vi "Update Message Setter.vi"(7 "RPC Message Name":string, 8 "error in (no error)":errorcluster, 10 "Message Getter in":refnum<vi>, 11 "RPC Messages Folder (ProjectItem) in":refnum<vi>) -> (0 "error out":errorcluster, 2 "Message Getter out":refnum<vi>, 3 "RPC Messages Folder (ProjectItem) out":refnum<vi>)   [LabVIEW 2019, in "gRPC Scripting Tools.lvlib"]
uses:
  gRPC Scripting Tools.lvlib
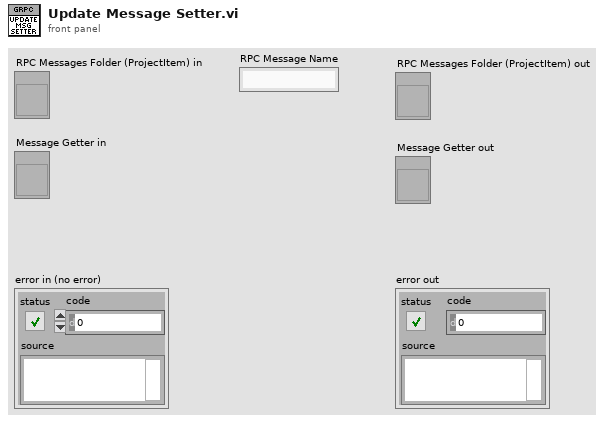
[diagram p1: front panel]
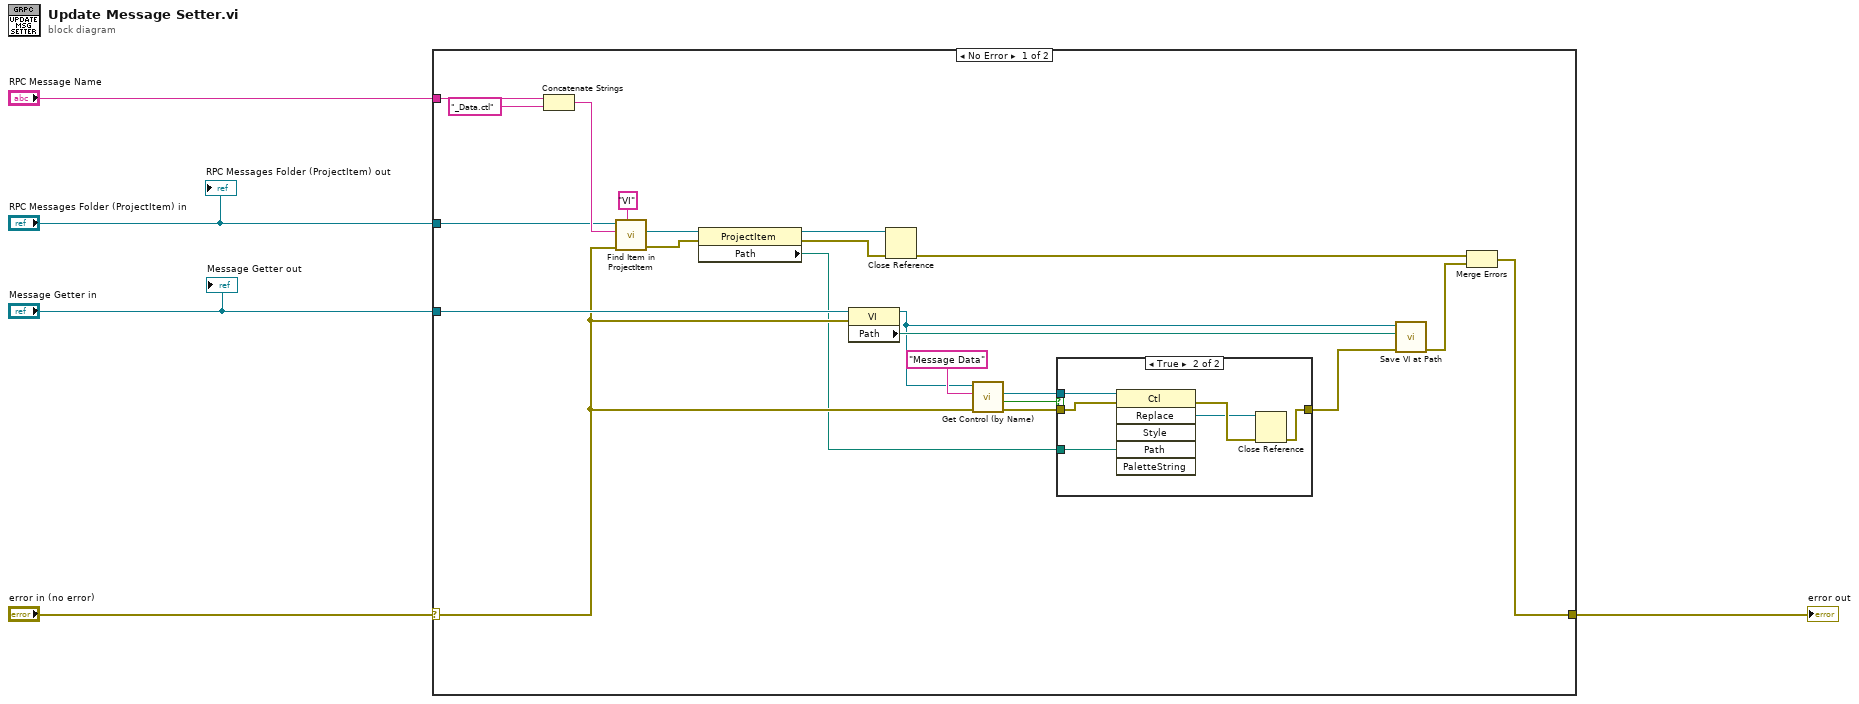
[diagram p0: block diagram]
diagram:
  n1 = case shown="No Error" "error in (no error)" {
    selector: "error in (no error)" -> [w8 w35]
    tunnel: "Message Getter in" -> [w26 _]
    tunnel: [w25 w35] -> w4
    tunnel: "RPC Message Name" -> [w16 _]
    tunnel: "RPC Messages Folder (ProjectItem) in" -> [w14 _]
    frame No Error {
      n2 = Concatenate Strings(w16, "_Data.ctl" ("string")) -> (w18:string)
      n3 = call "Find Item in ProjectItem.vi"("Item Type"="VI", "error in (no error)"=w8, "Name"=w18, "ProjectItem in"=w14) -> ("error out"=w20:errorcluster, "Item Refnum out"=w19:refnum<vi>)  [unwired: 4 in, 2 out]
      n4 = property class="ProjectItem"(reference=w19, error in=w20) -> (reference out=w21:refnum<vi>, error out=w22:errorcluster, "Path"=w6:path)
      n5 = property class="VI"(reference=w26, error in=w8) -> (reference out=w9:refnum<vi>, "Path"=w27:path)  [unwired: 1 out]
      n6 = Close Reference(reference=w21, error in (no error)=w22) -> (error out=w24:errorcluster)
      n7 = call "Get Control (by Name).vi"("error in (no error)"=w8, "Control Label"="Message Data" ("name/order"), "Owner VI in"=w9) -> ("error out"=w12:errorcluster, "Found ?"=w13:bool, "Control Refnum"=w11:refnum<vi>)  [unwired: 5 in, 1 out]
      n8 = case shown="True" w13 {
        tunnel: [w28 w34] -> w7
        tunnel: w11 -> [_ w31]
        tunnel: w12 -> [w28 w30]
        tunnel: w6 -> [_ w29]
        frame False {
        }
        frame True {
          n9 = invoke class="Ctl" method="Replace"(reference=w31, error in=w30, "Path"=w29) -> (error out=w33:errorcluster, "Replace"=w32:refnum<vi>)  [unwired: 3 in, 4 out]
          n10 = Close Reference(reference=w32, error in (no error)=w33) -> (error out=w34:errorcluster)
        }
      }
      n11 = call "Save VI at Path.vi"("error in (no error)"=w7, "Path"=w27, "VI in"=w9) -> ("error out"=w23:errorcluster)  [unwired: 6 in, 2 out]
      n12 = Merge Errors(w24, w23) -> (w25:errorcluster)
    }
    frame Error {
    }
  }
  "error out" <- w4
  "RPC Messages Folder (ProjectItem) out" <- "RPC Messages Folder (ProjectItem) in"
  "Message Getter out" <- "Message Getter in"
